vi "Mono Connect Test.vi"() -> ()   [LabVIEW 2015]
uses:
  K:/OSSIP/Optical Test Setup/System Qualification/LabVIEW Development/Cornerstone.dll
  Cornerstone.dll
panel:
  out "Mono Connection Status":bool=TRUE
  in  "error in (no error)":errorcluster
  out "error out":errorcluster
  out "CmdLib":refnum<k24>
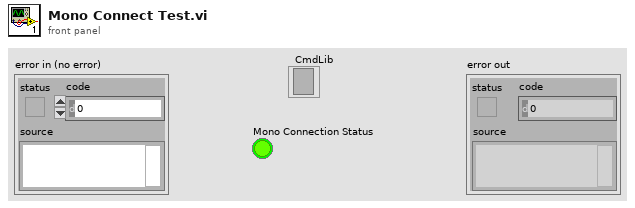
[diagram p1: front panel]
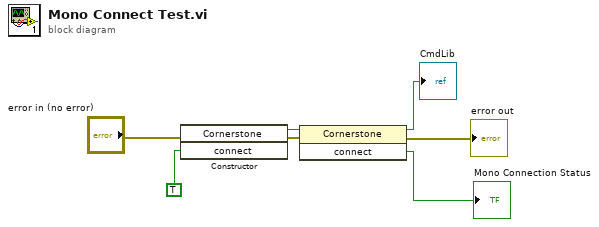
[diagram p0: block diagram]
diagram:
  n1 = constructor class="Cornerstone"(error in="error in (no error)", "connect"=TRUE) -> (reference out=w3:refnum<k24>, error out=w2:errorcluster)  [unwired: 2 in, 2 out]
  n2 = invoke class="Cornerstone" method="connect"(reference=w3, error in=w2) -> (reference out=→"CmdLib":refnum<k24>, error out=→"error out":errorcluster, "connect"=→"Mono Connection Status":bool)  [unwired: 1 in]
